vi "Error Write Watch.vi"(8 "error in":errorcluster, 10 "Watchdog STS":i32, 11 "Climate Chamber in":refnum<class "Climate Chamber.lvclass">) -> (0 "error out":errorcluster, 3 "Climate Chamber out":refnum<class "Climate Chamber.lvclass">)   [LabVIEW 2023, in "Climate Chamber.lvclass"]
uses:
  Climate Chamber.lvclass
  Climate Chamber.lvclass/Climate Chamber.ctl
  Low Level Capabilities/Error/Error.lvclass
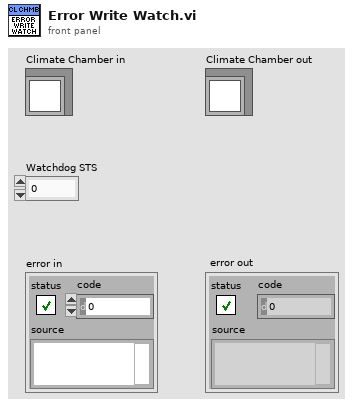
[diagram p1: front panel]
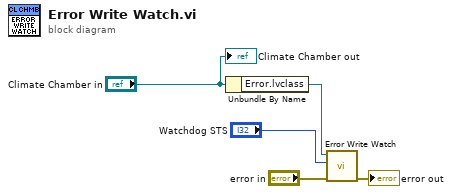
[diagram p0: block diagram]
diagram:
  n1 = Unbundle By Name("Climate Chamber in") -> ("Error.lvclass"=w2:refnum<class "Error.lvclass">)
  n2 = call-dynamic "Error Write Watch.vi"("error in"="error in", "Watchdog STS"="Watchdog STS", "Error in"=w2) -> ("error out"=→"error out":errorcluster)  [unwired: 7 in, 1 out]
  "Climate Chamber out" <- "Climate Chamber in"
